vi "ClusterwitharrayU8.vi"(1 "Cluster In":cluster{"Array In":u8[], "Numeric Input":u8}, 2 "Base":u8) -> (0 "Cluster Out":cluster{"Array Out":u8[], "Numeric Output":u8})   [LabVIEW 2013]
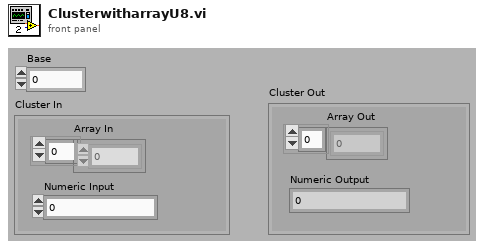
[diagram p1: front panel]
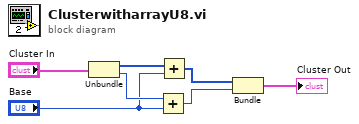
[diagram p0: block diagram]
diagram:
  n1 = Unbundle("Cluster In") -> ("Array In"=w7:u8[], "Numeric Input"=w6:u8)
  n2 = Add(x=w6, y="Base") -> (x+y=w4:u8)
  n3 = Add(x=w7, y="Base") -> (x+y=w5:u8[])
  n4 = Bundle(w5, w4) -> (→"Cluster Out":cluster{u8[], u8})  [unwired: 1 out]
